vi "Output to Motor.vi"(8 "error in (no error)":errorcluster, 9 "Fast Loop State in":T1, 11 "IMU_sample_rate":i32=200) -> (0 "error out":errorcluster, 4 "Fast Loop State out":T1)   [LabVIEW 2014]
uses:
  <userlib>/UCSD Robotics Lab/Robotics-Cape/LV/libroboticscape.lvlib
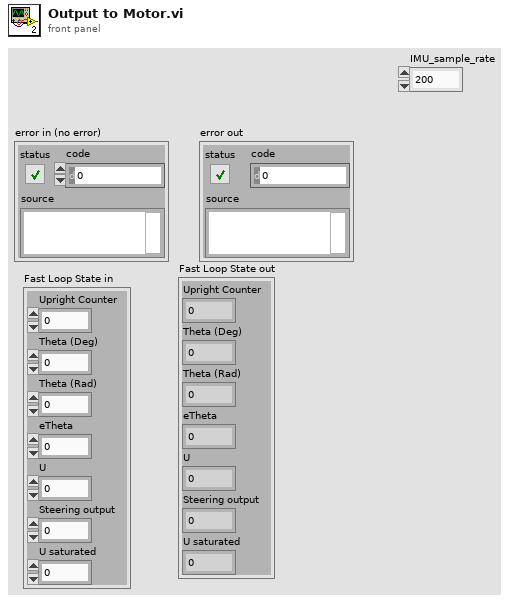
[diagram p1: front panel]
types:
  T1 = cluster{"Upright Counter":dbl, "Theta (Deg)":dbl, "Theta (Rad)":dbl, "eTheta":dbl, "U":dbl, "Steering output":dbl, "U saturated":sgl}
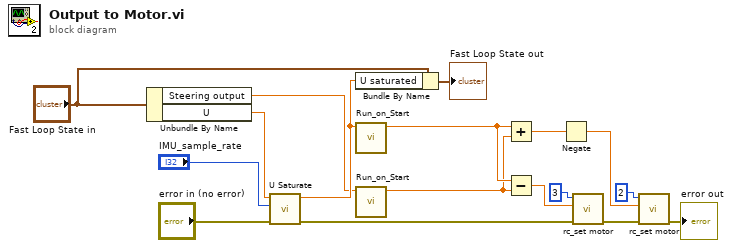
[diagram p0: block diagram]
diagram:
  n1 = Unbundle By Name("Fast Loop State in") -> ("Steering output"=w2:dbl, "U"=w3:dbl)
  n2 = call "U Saturate.vi"("error in (no error)"="error in (no error)", "IMU_sample_rate"="IMU_sample_rate", "Filtered x"=w3) -> ("error out"=w11:errorcluster, "val out"=w6:sgl)  [unwired: 7 in]
  n3 = Bundle By Name(cluster="Fast Loop State in", "U saturated"=w6) -> (→"Fast Loop State out":T1)
  n4 = call "Run_on_Start.vi"("val in"=w6) -> ("Val out"=w9:sgl)  [unwired: 10 in]
  n5 = call "Run_on_Start.vi"("val in"=w2) -> ("Val out"=w8:sgl)  [unwired: 10 in]
  n6 = Add(x=w9, y=w8) -> (x+y=w7:sgl)
  n7 = Subtract(x=w9, y=w8) -> (x-y=w10:sgl)
  n8 = Negate(x=w7) -> (-x=w15:sgl)
  n9 = call <userlib>:"rc_set motor.vi"("error in (no error)"=w11, "duty"=w10, "motor"=3) -> ("error out"=w16:errorcluster)  [unwired: 7 in, 1 out]
  n10 = call <userlib>:"rc_set motor.vi"("error in (no error)"=w16, "duty"=w15, "motor"=2) -> ("error out"=→"error out":errorcluster)  [unwired: 7 in, 1 out]
